vi "Component Loader.Load.Packed Library.Classes.vi"(8 "error in (no error)":errorcluster, 10 "packed library name":string, 11 "Component Loader in":refnum<class "Component Loader.lvclass">) -> (0 "error out":errorcluster, 2 "objects":refnum<class>[](array[class]), 3 "Component Loader out":refnum<class "Component Loader.lvclass">)   [LabVIEW 2017, in "DSF.Engine.lvlib" / "Component Loader.lvclass"]
uses:
  Component Loader.lvclass
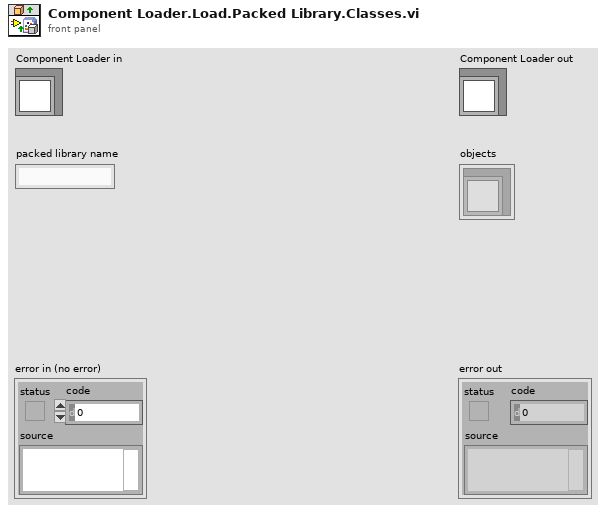
[diagram p1: front panel]
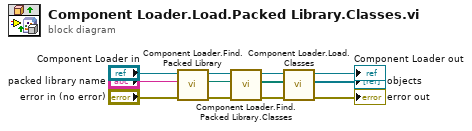
[diagram p0: block diagram]
diagram:
  n1 = call "Component Loader.Find.Packed Library.vi"("error in (no error)"="error in (no error)", "packed library name"="packed library name", "Component Loader in"="Component Loader in") -> ("error out"=w7:errorcluster, "packed library path"=w9:path, "Component Loader out"=w8:refnum<class "Component Loader.lvclass">)  [unwired: 6 in]
  n2 = call "Component Loader.Find.Packed Library.Classes.vi"("error in (no error)"=w7, "packed library path"=w9, "Component Loader in"=w8) -> ("error out"=w5:errorcluster, "class paths"=w4:path[], "Component Loader out"=w6:refnum<class "Component Loader.lvclass">)  [unwired: 6 in]
  n3 = call "Component Loader.Load.Classes.vi"("error in (no error)"=w5, "class paths"=w4, "Component Loader in"=w6) -> ("error out"=→"error out":errorcluster, "objects"=→"objects":refnum<class>[], "Component Loader out"=→"Component Loader out":refnum<class "Component Loader.lvclass">)  [unwired: 6 in]
